vi "User Query COMs.vi"(11 "COMs":refnum<visa-resource-name>[](array[refnum])) -> (3 "Selected COM":refnum<visa-resource-name>)   [LabVIEW 2020, in "DLP Design Modules Driver.lvlib"]
uses:
  DLP Design Modules Driver.lvlib
panel:
  in  "Tab Control":enum32{"User", "Back Params"}(tab)
  in  "Detected Device COMs":u16(ring) items=["COM4", "COM32"]
  out "UserMsg":string
  in  "Select  Button":bool
  in  "Device Type":enum16{"IOR4 device", "IO20 device"}(ring)
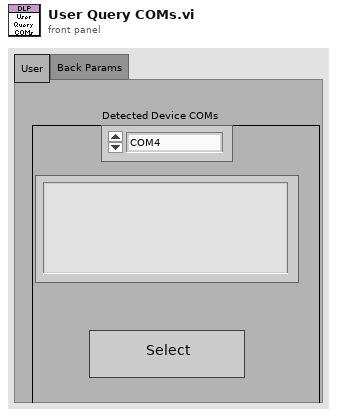
[diagram p1: front panel]
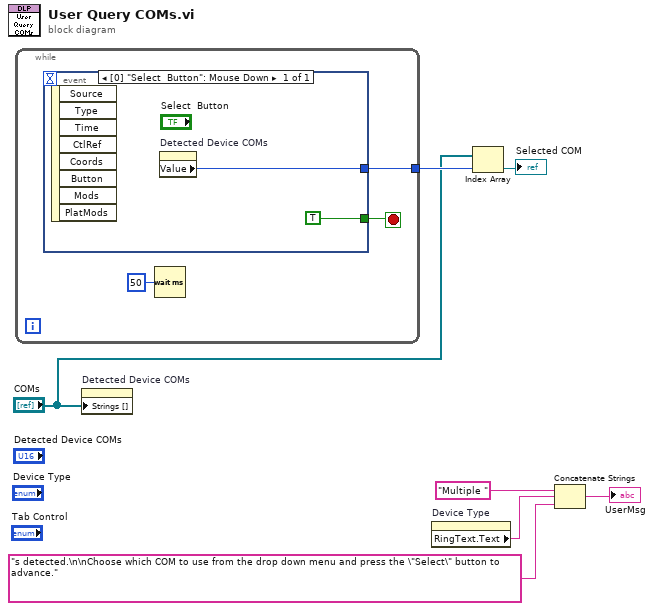
[diagram p0: block diagram]
diagram:
  n1 = while {
    tunnel: [w10] -> w3
    stop <- w8 stop-if-true
    n2 = event shown="[0] \"Select  Button\": Mouse Down" {
      selector: _ -> [_]
      dyn-events: _ -> [_]
      timeout: _ -> [_]
      tunnel: [w12] -> w10
      tunnel: [TRUE] -> w8
      event "Select  Button": Mouse Down {
        n3 = event-data() -> ()  [unwired: 1 in, 8 out]
        n4 = property on="Detected Device COMs" class="Ring (strict)"() -> ("Value"=w12:u16)  [unwired: 2 in, 2 out]
      }
    }
    n5 = Wait (ms)(milliseconds to wait=u32 50) -> ()  [unwired: 1 out]
  }
  n6 = property on="Detected Device COMs" class="Ring (strict)"("Strings []"="COMs") -> ()  [unwired: 2 in, 2 out]
  n7 = property on="Device Type" class="Enum (strict)"() -> ("RingText.Text"=w5:string)  [unwired: 2 in, 2 out]
  n8 = Index Array(array="COMs", index=w3) -> (element=→"Selected COM":refnum<visa-resource-name>)
  n9 = Concatenate Strings("Multiple ", w5, "s detected.\n\nChoose which COM to use from the drop down menu and press the \"Select\" button to advance.") -> (→"UserMsg":string)
